vi "Plot Maximize Button.vi"(7 "VI ref":refnum<vi>, 8 "error in (no error)":errorcluster, 9 "max button reference":refnum<vi>, 10 "Maximize?":bool, 11 "StokePlotHandle in":refnum<class "BjusticePlotHandle.lvclass">) -> (0 "error out":errorcluster, 3 "StokePlotHandle out":refnum<class "BjusticePlotHandle.lvclass">)   [LabVIEW 2021, in "BjusticePlotHandle.lvclass"]
uses:
  BjusticePlotHandle.lvclass
  1PLOT to MPLOT UE.ctl
  1PLOT to MPLOT type.ctl
  Maximize action.ctl
  BjusticePlotHandle.lvclass/BjusticePlotHandle.ctl
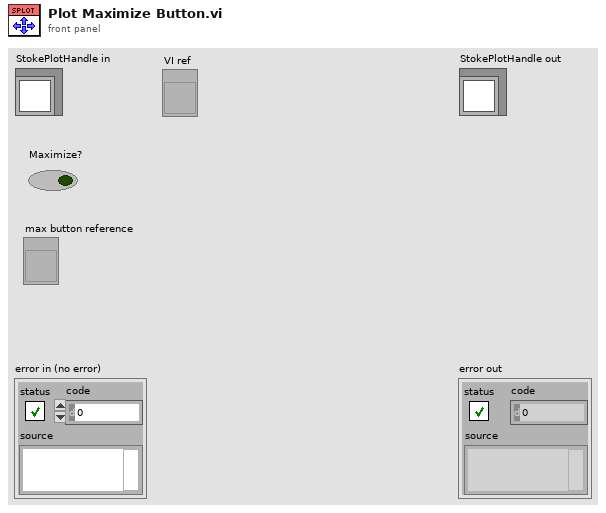
[diagram p1: front panel]
types:
  T1 = typedef "BjusticePlotHandle.lvclass/Maximize action.ctl" = cluster{"Maximize?":bool, "max button":refnum<vi>}
  T2 = typedef "BjusticePlotHandle.lvclass/1PLOT to MPLOT type.ctl" = enum16{"Maximize", "ShortcutMenu"}
  T3 = typedef "BjusticePlotHandle.lvclass/1PLOT to MPLOT UE.ctl" = cluster{"Type":T2, "source VI ref":refnum<vi>, "data":variant}
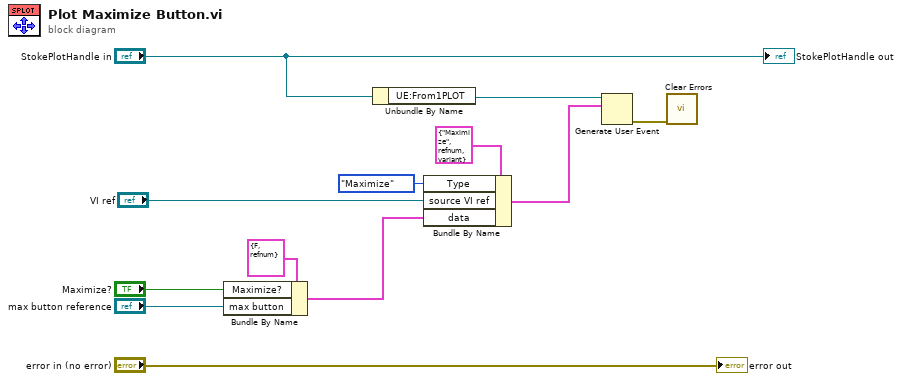
[diagram p0: block diagram]
diagram:
  n1 = Bundle By Name(cluster=T1 {"Maximize?"=FALSE, "max button"=refnum} ("Cluster"), "Maximize?"="Maximize?", "max button"="max button reference") -> (w2:T1)
  n2 = Unbundle By Name("StokePlotHandle in") -> ("UE:From1PLOT"=w12:refnum<user-event>)
  n3 = Bundle By Name(cluster=T3 {"Type"=enum."Maximize", "source VI ref"=refnum, "data"=variant(string "")} ("event data"), "Type"=1PLOT_to_MPLOT_type."Maximize", "source VI ref"="VI ref", "data"=w2) -> (w9:T3)
  n4 = Generate User Event(user event=w12, event data cluster=w9) -> (error out=w11:errorcluster)  [unwired: 2 in, 1 out]
  n5 = call <vilib>:"Clear Errors.vi"("error in (no error)"=w11) -> ()  [unwired: 5 in, 2 out]
  "error out" <- "error in (no error)"
  "StokePlotHandle out" <- "StokePlotHandle in"
